vi "Skip.vi"(7 "Description":string, 8 "error in (no error)":errorcluster, 9 "Message":string, 11 "LUnit Test Case In":refnum<class "LUnit Test Case.lvclass">) -> (0 "error out":errorcluster, 3 "LUnit Test Case Out":refnum<class "LUnit Test Case.lvclass">)   [LabVIEW 2020, in "LUnit Test Case.lvclass"]
doc: "Ignores results from the calling test method when evaluating the test case result. A description and message may be provided."
uses:
  LUnit Test Case.lvclass
  Result Types/Assertion Result/Public/TypeDefs/Assertion Type.ctl
  Result Types/Assertion Result/Assertion Result.lvlib
  Result Types/Assertion Result/Public/TypeDefs/Status.ctl
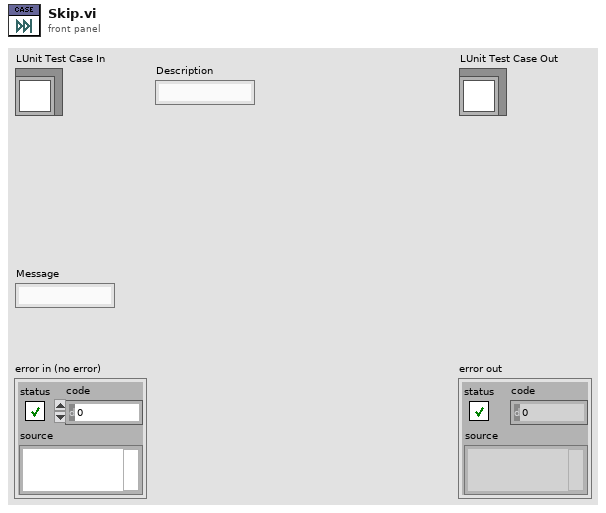
[diagram p1: front panel]
types:
  T1 = typedef "Assertion Result.lvlib/Status.ctl" = enum16{"Pass", "Fail", "Error", "Skipped", "Setup Error", "Broken", "Teardown Error"}
  T2 = typedef "Assertion Result.lvlib/Assertion Type.ctl" = enum16{"None", "Pass", "Fail", "Skip", "Pass if Equal", "Fail if Equal", "Pass if Error", "Fail if Error", "Pass if", "Fail if"}
  T3 = typedef "Assertion Result.lvlib/Assertion Result.ctl" = cluster{"Status":T1, "Message":string, "Description":string, "Assertion Type":T2}
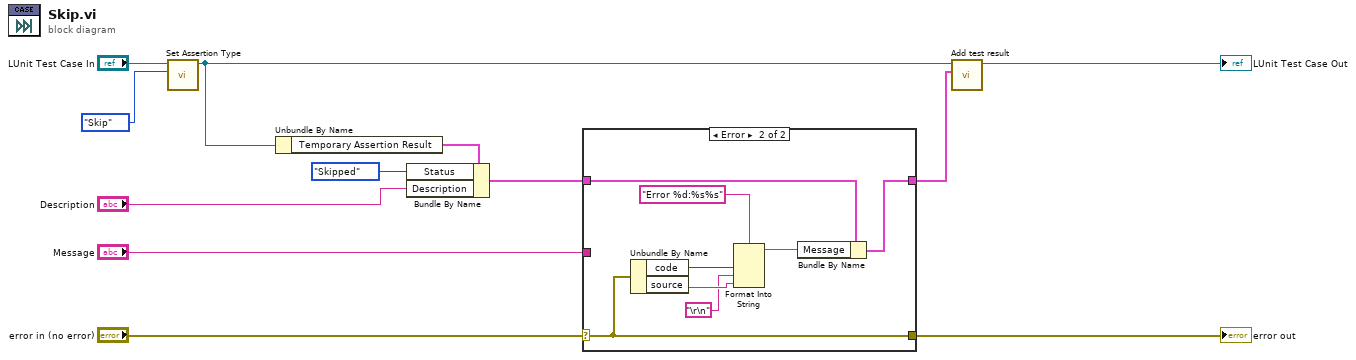
[diagram p0: block diagram]
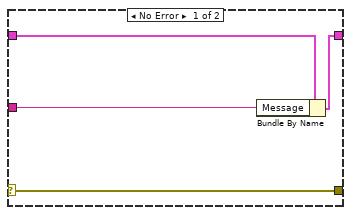
[diagram p2: hidden frame]
diagram:
  n1 = call "Set Assertion Type.vi"("Assertion Type"=Assertion_Type."Skip", "LUnit Test Case In"="LUnit Test Case In") -> ("LUnit Test Case Out"=w9:refnum<class "LUnit Test Case.lvclass">)  [unwired: 9 in]
  n2 = Unbundle By Name(w9) -> ("Temporary Assertion Result"=w6:T3)
  n3 = Bundle By Name(cluster=w6, "Status"=Status."Skipped", "Description"="Description") -> (w2:T3)
  n4 = case shown="Error" "error in (no error)" {
    selector: "error in (no error)" -> [w16 w23]
    tunnel: [w16 w23] -> w8
    tunnel: [w14 w24] -> w1
    tunnel: "Message" -> [w15 _]
    tunnel: w2 -> [w13 w17]
    frame No Error {
      n5 = Bundle By Name(cluster=w13, "Message"=w15) -> (w14:T3)
    }
    frame Error {
      n6 = Unbundle By Name(w23) -> ("code"=w21:i32, "source"=w19:string)
      n7 = Format Into String(format string="Error %d:%s%s", w21, "\r\n", w19) -> (resulting string=w20:string)  [unwired: 2 in, 1 out]
      n8 = Bundle By Name(cluster=w17, "Message"=w20) -> (w24:T3)
    }
  }
  "error out" <- w8
  n9 = call "Add test result.vi"("Test Result"=w1, "LUnit Test Case In"=w9) -> ("LUnit Test Case Out"=→"LUnit Test Case Out":refnum<class "LUnit Test Case.lvclass">)  [unwired: 9 in]
